vi "[Global]Mask.vi"() -> ()   [LabVIEW 2015]
panel:
  out "Mask":string[](array[string])=["ExtractedImage0", "ExtractedImage1", "ExtractedImage2", "ExtractedImage3", "ExtractedImage4", "ExtractedImage5", "ExtractedImage6", "ExtractedImage7"]
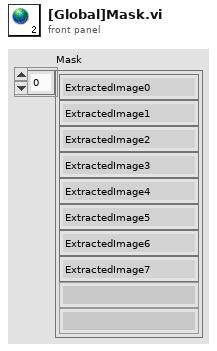
[diagram p1: front panel]
diagram:
